vi "STM Multi-Client - Server (RT).vi"() -> ()   [LabVIEW 2019]
uses:
  <vilib>/NI/STM/Connection Manager/TCP/TCP Connection Method.ctl
  <vilib>/NI/STM/SubVIs/MetaDataElement.ctl
  <vilib>/Platform/TimedLoop/XDataNode/timing_clust.ctl
  <vilib>/Platform/TimedLoop/XDataNode/nitl_modes.ctl
  <vilib>/Platform/TimedLoop/XDataNode/wakeup.ctl
  <vilib>/NI/STM/TCP/Write Meta Data (TCP Ref).vi
  <vilib>/NI/STM/TCP/Read Message (TCP).vi
  <vilib>/NI/STM/TCP/Write Message (TCP).vi
  <vilib>/NI/STM/TCP/Write Meta Data (TCP Clst).vi
  <vilib>/platform/TimedLoop/XDataNode/XDataNode.xnode
  <vilib>/Platform/TimedLoop/XDataNode/XDNodeRunTimeDep.lvlib
  <vilib>/real-time/NI_Real-Time Libraries.lvlib
  <vilib>/NI/STM/NI STM.lvlib
panel:
  out "Numeric 4":i32
  out "Numeric 3":i32
  out "Numeric 2":i32
  out "Numeric":i32
  in  "Stop non-critical loops":bool
  out "error out":errorcluster
  out "Number of \nConnections":i32
  # "Overview: Demonstrate the use of the STM library to implement a Single Server Multi Client application design. \nRequirements: LabVIEW Full Development System, STM Library version 3.x or later\nInstructions: \n1. Run the STM Multi-Client - Server (RT) VI\n2. Set the Target IP Address in the STM Multi-Client - Client VI to match the IP address of the server\n3. Run the STM Multi-Client - Client VI\n4. Change the Channel to choose between four different waveform"
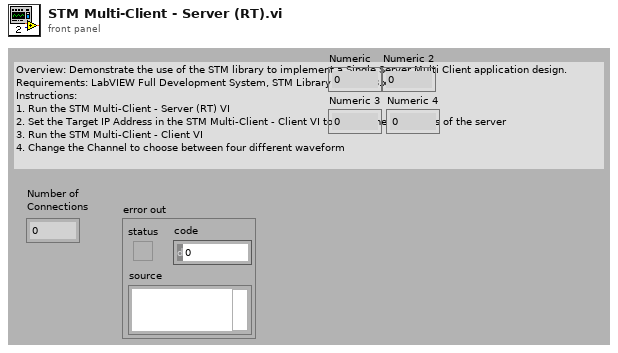
[diagram p1: front panel]
types:
  T1 = typedef "NI STM.lvlib/MetaDataElement.ctl" = string
  T2 = typedef "NI STM.lvlib/TCP Connection Method.ctl" = enum16{"Initialize", "Add Connection", "Set Properties", "Get Connection(s)", "Remove Connection", "Remove All Connections", "Get Connection Count"}
  T3 = typedef "RT FIFOs (STM Multi-Client).ctl" = cluster{"Data FIFO":T4, "Stop FIFO":T5}
  T4 = typedef "NI_Real-Time Libraries.lvlib/RTFIFORefnum DBLA.ctl" = cluster{"index":u32, "id":u32, "type":dbl[], "size":u32}
  T5 = typedef "NI_Real-Time Libraries.lvlib/RTFIFORefnum BOOL.ctl" = cluster{"index":u32, "id":u32, "type":bool, "size":u32}
  T6 = typedef "XDNodeRunTimeDep.lvlib/timing_clust.ctl" = cluster{"Expected End [f-1]":u64, "Actual End [f-1]":u64, "Finished Late? [f-1]":bool, "Expected End [i-1]":u64, "Actual End [i-1]":u64, "Finished Late? [i-1]":bool, "Expected Start [i]":u64, "Actual Start [i]":u64, "Expected Start [f]":u64, "Actual Start [f]":u64, "Source Name":string, "Structure Name":string, "Period":i64, "Deadline":i64, "Offset":i64, "Start":i64, "Priority":i32, "Timeout":i32, "Mode":T7, "Wakeup Reason":T8, "Error":errorcluster, "Source Type":string, "Secondary Source Type":string, "Global End Time":u64, "Global Start Time":u64, "Frame Duration":u64, "Iteration Duration":u64, "Assigned CPU":i32, "I/O Scan Engine Mode":u32}
  T7 = typedef "XDNodeRunTimeDep.lvlib/nitl_modes.ctl" = enum32{"No Change", "Process missed periods, maintain original phase", "Discard missed periods, maintain original phase", "Process missed periods, ignore original phase", "Discard missed periods, ignore original phase"}
  T8 = typedef "XDNodeRunTimeDep.lvlib/wakeup.ctl" = enum32{"Normal", "Aborted", "Asynchronous wakeup", "Timing source error", "Timed loop error", "Timeout"}
  T9 = typedef "NI STM.lvlib/TCP Connection Info.ctl" = cluster{"connection ID":refnum<k5>, "meta data":T1[]}
  T10 = typedef "NI STM.lvlib/TCP Connection Properties.ctl" = cluster{"Name":string, "Address":string, "Custom":string}
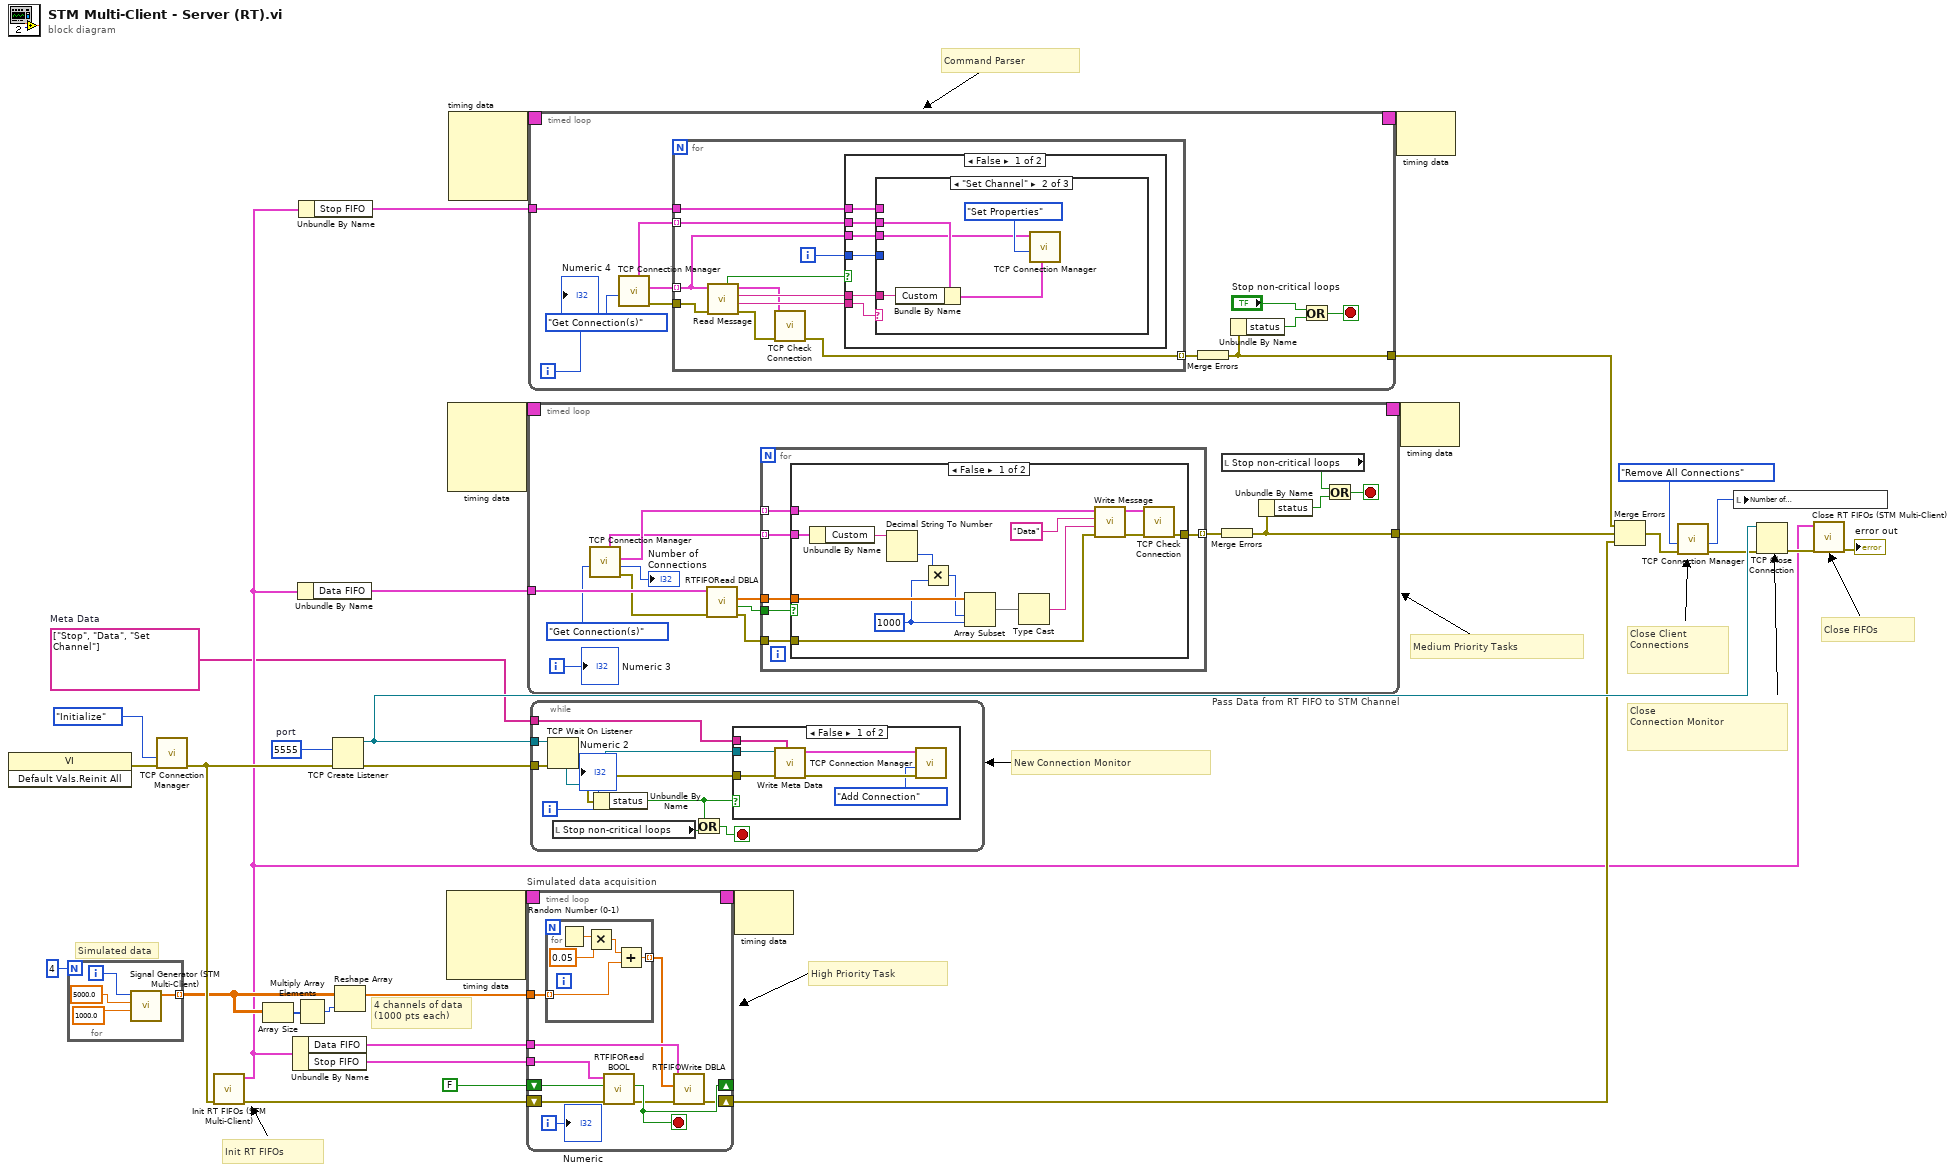
[diagram p0: block diagram]
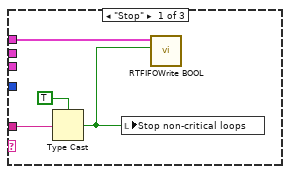
[diagram p3: hidden frame]
diagram:
  w1 = T1[] ["Stop", "Data", "Set Channel"]  # Meta Data
  w31 = u16 5555  # port
  # "4 channels of data\n(1000 pts each)"
  # "Command Parser"
  # "Medium Priority Tasks"
  # "Close \nConnection Monitor"
  # "Init RT FIFOs"
  # "Simulated data"
  # "New Connection Monitor"
  # "Close Client\nConnections"
  # "Close FIFOs"
  # "High Priority Task"
  n1 = invoke class="VI" method="Default Vals.Reinit All"() -> (error out=w7:errorcluster)  [unwired: 3 in, 2 out]
  n2 = for {
    N: 4 -> [_]
    tunnel: [w37] -> w17 mode=indexing
    i -> [w38]
    n3 = call "Signal Generator (STM Multi-Client).vi"("#Samples"=1000.0, "frequency"=5000.0, "Signal Type"=w38) -> ("Data"=w37:dbl[])  [unwired: 7 in, 1 out]
  }
  n4 = call <vilib>:"TCP Connection Manager.vi"("error in"=w7, "method"=TCP_Connection_Method."Initialize") -> ("error out"=w29:errorcluster)  [unwired: 4 in, 5 out]
  n5 = call "Init RT FIFOs (STM Multi-Client).vi"("error in (no error)"=w29) -> ("error out"=w10:errorcluster, "FIFOs out"=w8:T3)  [unwired: 9 in]
  n6 = Array Size(array=w17) -> (size(s)=w16:i32[])
  n7 = Unbundle By Name(w8) -> ("Data FIFO"=w12:T4, "Stop FIFO"=w13:T5)
  n8 = Multiply Array Elements(1:w16) -> (0:w15:i32)
  n9 = Unbundle By Name(w8) -> ("Data FIFO"=w27:T4)
  n10 = Unbundle By Name(w8) -> ("Stop FIFO"=w26:T5)
  n11 = TCP Create Listener(8:w29, 10:w31) -> (0:w32:errorcluster, 3:w30:refnum<k5>)  [unwired: 3 in, 1 out]
  n12 = Reshape Array(w17, w15) -> (w14:dbl[])
  n13 = node-c288() -> (w20:T6)  [unwired: 4 in]
  n14 = node-c288() -> (w22:T6)  [unwired: 4 in]
  n15 = node-c288() -> (w24:T6)  [unwired: 4 in]
  n16 = timed-loop "Simulated data acquisition" {
    tunnel: w14 -> [w41]
    tunnel: w13 -> [w48]
    tunnel: w12 -> [w44]
    shift-right: [w46] -> _
    shift-left: FALSE -> [w47]
    timing: w20 -> [_]
    timing-out: [_] -> w19
    shift-right: [w42] -> w9
    shift-left: w10 -> [w45]
    i -> [w39]
    stop <- w46 stop-if-true
    n17 = for {
      tunnel: w41 -> [w50] mode=indexing
      tunnel: [w49] -> w40 mode=indexing
      n18 = Random Number (0-1)() -> (number: 0 to 1=w53:dbl)
      n19 = Multiply(x=w53, y=0.05) -> (x*y=w51:dbl)
      n20 = Add(x=w51, y=w50) -> (x+y=w49:dbl)
    }
    n21 = call <vilib>:"RTFIFORead BOOL.vi"("error in (no error)"=w45, "element"=w47, "rt fifo"=w48) -> ("error out"=w43:errorcluster, "element out"=w46:bool)  [unwired: 5 in, 2 out]
    n22 = call <vilib>:"RTFIFOWrite DBLA.vi"("error in (no error)"=w43, "element"=w40, "rt fifo"=w44) -> ("error out"=w42:errorcluster)  [unwired: 6 in, 2 out]
    "Numeric" <- w39
  }
  n23 = timed-loop "Pass Data from RT FIFO to STM Channel" {
    tunnel: [w64] -> w34
    tunnel: w27 -> [w62]
    timing: w22 -> [_]
    timing-out: [_] -> w21
    i -> [w56]
    stop <- w70 stop-if-true
    n24 = call <vilib>:"TCP Connection Manager.vi"("method"=TCP_Connection_Method."Get Connection(s)") -> ("error out"=w58:errorcluster, "number of connections"=→"Number of \nConnections":i32, "all connections"=w67:T9[], "all properties"=w63:T10[])  [unwired: 5 in, 2 out]
    n25 = call <vilib>:"RTFIFORead DBLA.vi"("error in (no error)"=w58, "rt fifo"=w62) -> ("error out"=w57:errorcluster, "empty"=w60:bool, "element out"=w61:dbl[])  [unwired: 6 in, 1 out]
    n26 = for {
      tunnel: [w75] -> w66 mode=indexing
      tunnel: w67 -> [w76] mode=indexing
      tunnel: w63 -> [w74] mode=indexing
      tunnel: w61 -> [w73]
      tunnel: w60 -> [w72]
      tunnel: w57 -> [w71]
      n27 = case shown="False" w72 {
        tunnel: w76 -> [w79 _]
        tunnel: [w88 _] -> w75
        tunnel: w73 -> [w86 _]
        tunnel: w74 -> [w85 _]
        tunnel: w71 -> [w77 _]
        frame False {
          w84 = 1000 ("length")
          n28 = Unbundle By Name(w85) -> ("Custom"=w83:string)
          n29 = Decimal String To Number(string=w83) -> (number=w80:i32)  [unwired: 2 in, 1 out]
          n30 = Multiply(x=w80, y=w84) -> (x*y=w82:i32)
          n31 = Array Subset(array=w86, index=w82, length=w84) -> (w81:dbl[])
          n32 = Type Cast(x=w81) -> (*(type *) &x=w87:string)  [unwired: 1 in]
          n33 = call-poly <vilib>:"Write Message.vi"("error in"=w77, "data"=w87, "name"="Data" ("Name"), "connection info in"=w79) -> ("error out"=w89:errorcluster, "connection info out"=w78:T9)  [unwired: 6 in]
          n34 = call <vilib>:"TCP Check Connection.vi"("error in"=w89, "connection in"=w78) -> ("error out"=w88:errorcluster)  [unwired: 7 in, 2 out]
        }
        frame True {
        }
      }
    }
    n35 = local read "Stop non-critical loops"() -> (w68:bool)
    n36 = Merge Errors(w66) -> (w64:errorcluster)
    n37 = Unbundle By Name(w64) -> ("status"=w69:bool)
    n38 = Or(x=w68, y=w69) -> (x .or. y?=w70:bool)
    "Numeric 3" <- w56
  }
  n39 = timed-loop {
    tunnel: [w100] -> w33
    tunnel: w26 -> [w98]
    timing: w24 -> [_]
    timing-out: [_] -> w23
    i -> [w93]
    stop <- w103 stop-if-true
    n40 = call <vilib>:"TCP Connection Manager.vi"("method"=TCP_Connection_Method."Get Connection(s)") -> ("error out"=w94:errorcluster, "all connections"=w99:T9[], "all properties"=w97:T10[])  [unwired: 5 in, 3 out]
    n41 = for {
      tunnel: [w110] -> w101 mode=indexing
      tunnel: w99 -> [w105] mode=indexing
      tunnel: w98 -> [w109]
      tunnel: w97 -> [w107] mode=indexing
      tunnel: w94 -> [w104]
      i -> [w108]
      n42 = call-poly <vilib>:"Read Message.vi"("error in"=w104, "connection info in"=w105) -> ("error out"=w111:errorcluster, "name"=w114:T1, "data string"=w113:string, "connection info out"=w106:T9, "timed out?"=w112:bool)  [unwired: 4 in, 1 out]
      n43 = call <vilib>:"TCP Check Connection.vi"("error in"=w111, "connection in"=w106) -> ("error out"=w110:errorcluster)  [unwired: 7 in, 2 out]
      n44 = case shown="False" w112 {
        tunnel: w114 -> [w115 _]
        tunnel: w113 -> [w120 _]
        tunnel: w109 -> [w119 _]
        tunnel: w105 -> [w118 _]
        tunnel: w108 -> [w117 _]
        tunnel: w107 -> [w116 _]
        frame False {
          n45 = case shown="\"Set Channel\"" w115 {
            tunnel: w120 -> [w124 w125 _]
            tunnel: w119 -> [w121 _ _]
            tunnel: w118 -> [_ w126 _]
            tunnel: w117 -> [_ _ _]
            tunnel: w116 -> [_ w129 _]
            frame "Stop" {
              n46 = Type Cast(type=TRUE, x=w124) -> (*(type *) &x=w122:bool)
              n47 = local write "Stop non-critical loops"(w122) -> ()
              n48 = call <vilib>:"RTFIFOWrite BOOL.vi"("element"=w122, "rt fifo"=w121) -> ()  [unwired: 7 in, 3 out]
            }
            frame "Set Channel" {
              n49 = Bundle By Name(cluster=w129, "Custom"=w125) -> (w128:T10)
              n50 = call <vilib>:"TCP Connection Manager.vi"("properties in"=w128, "method"=TCP_Connection_Method."Set Properties", "connection in"=w126) -> ()  [unwired: 3 in, 6 out]
            }
            frame Default {
            }
          }
        }
        frame True {
        }
      }
    }
    n51 = Merge Errors(w101) -> (w100:errorcluster)
    n52 = Unbundle By Name(w100) -> ("status"=w102:bool)
    n53 = Or(x="Stop non-critical loops", y=w102) -> (x .or. y?=w103:bool)
    "Numeric 4" <- w93
  }
  n54 = while "Listen loop.  Append new connections to a synchronized queue." {
    tunnel: w30 -> [w139]
    tunnel: w32 -> [w140]
    tunnel: w1 -> [w136]
    i -> [w132]
    stop <- w134 stop-if-true
    n55 = TCP Wait On Listener(8:w140, 11:w139) -> (0:w135:errorcluster, 4:w138:refnum<k5>)  [unwired: 2 in, 3 out]
    n56 = local read "Stop non-critical loops"() -> (w133:bool)
    n57 = Unbundle By Name(w135) -> ("status"=w137:bool)
    n58 = Or(x=w137, y=w133) -> (x .or. y?=w134:bool)
    n59 = case shown="False" w137 {
      tunnel: w138 -> [w146 _]
      tunnel: w136 -> [w141 _]
      tunnel: w135 -> [w144 _]
      frame False {
        n60 = call-poly <vilib>:"Write Meta Data.vi"("meta data"=w141, "error in"=w144, "connection ID"=w146) -> ("error out"=w145:errorcluster, "connection info out"=w142:T9)  [unwired: 7 in]
        n61 = call <vilib>:"TCP Connection Manager.vi"("error in"=w145, "method"=TCP_Connection_Method."Add Connection", "connection in"=w142) -> ()  [unwired: 3 in, 6 out]
      }
      frame True {
      }
    }
    "Numeric 2" <- w132
  }
  n62 = node-c288(w19) -> ()  [unwired: 1 out]
  n63 = node-c288(w23) -> ()  [unwired: 1 out]
  n64 = node-c288(w21) -> ()  [unwired: 1 out]
  n65 = Merge Errors(w33, w34, w9) -> (w6:errorcluster)
  n66 = call <vilib>:"TCP Connection Manager.vi"("error in"=w6, "method"=TCP_Connection_Method."Remove All Connections") -> ("error out"=w5:errorcluster, "number of connections"=w4:i32)  [unwired: 4 in, 4 out]
  n67 = local write "Number of \nConnections"(w4) -> ()
  n68 = TCP Close Connection(connection ID=w30, error in (no error)=w5) -> (error out=w28:errorcluster)  [unwired: 1 in, 1 out]
  n69 = call "Close RT FIFOs (STM Multi-Client).vi"("error in (no error)"=w28, "FIFOs In"=w8) -> ("error out"=→"error out":errorcluster)  [unwired: 9 in]
